vi "Create ARINC 429 Word (U32) from Label (U8).vi"(11 "label":u8 format="%03o") -> (3 "initial word":u32 format="%032b")   [LabVIEW 2020]
uses:
  51f8d117-4d3b-42bd-8ccb-0fcd1ffcafe8.vi
  51f8d117-4d3b-42bd-8ccb-0fcd1ffcafe8.vi/a7fcce85-1f75-4572-aeaa-ddfd463a7c5f.vi
panel:
  # "P (1) | SSM (2) | Parameter (19) | SDI (2) | LABEL (8)"
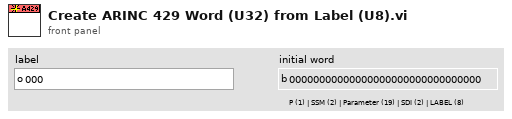
[diagram p1: front panel]
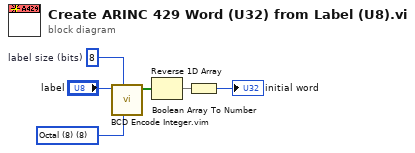
[diagram p0: block diagram]
diagram:
  w3 = 8  # label size (bits)
  w6 = u8 8 items=["Binary (2)"=2, "Octal (8)"=8, "Decimal (10)"=10, "Hexadecimal (16)"=16] ("base")
  n1 = call "BCD Encode Integer.vim"("base"=w6, "data size (bits)"=w3, "integer"="label") -> ("BCD encoded value"=w5:bool[])  [unwired: 7 in, 1 out]
  n2 = Reverse 1D Array(array=w5) -> (reversed array=w4:bool[])
  n3 = Boolean Array To Number(Boolean array=w4) -> (number=→"initial word":u32)
